vi "Tag Lookup_By Name.vi"(6 "Namespace":string, 8 "error in (no error)":errorcluster, 10 "Name":string) -> (0 "error out":errorcluster, 1 "found":bool, 2 "Tag Ref out":refnum<data-value>)   [LabVIEW 2020, in "Tag Engine Core.lvlib" / "Tag Core.lvclass"]
doc: "_SubVI_"
uses:
  Tag Core.lvclass
  Tag/Tag.lvclass
  Tag Core.lvclass/Tag Core.ctl
  <vilib>/Utility/error.llb/Error Cluster From Error Code.vi
  <vilib>/ErrorRing/Error Ring.xnode
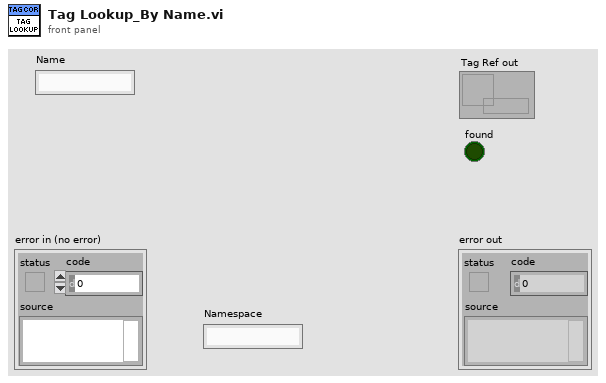
[diagram p1: front panel]
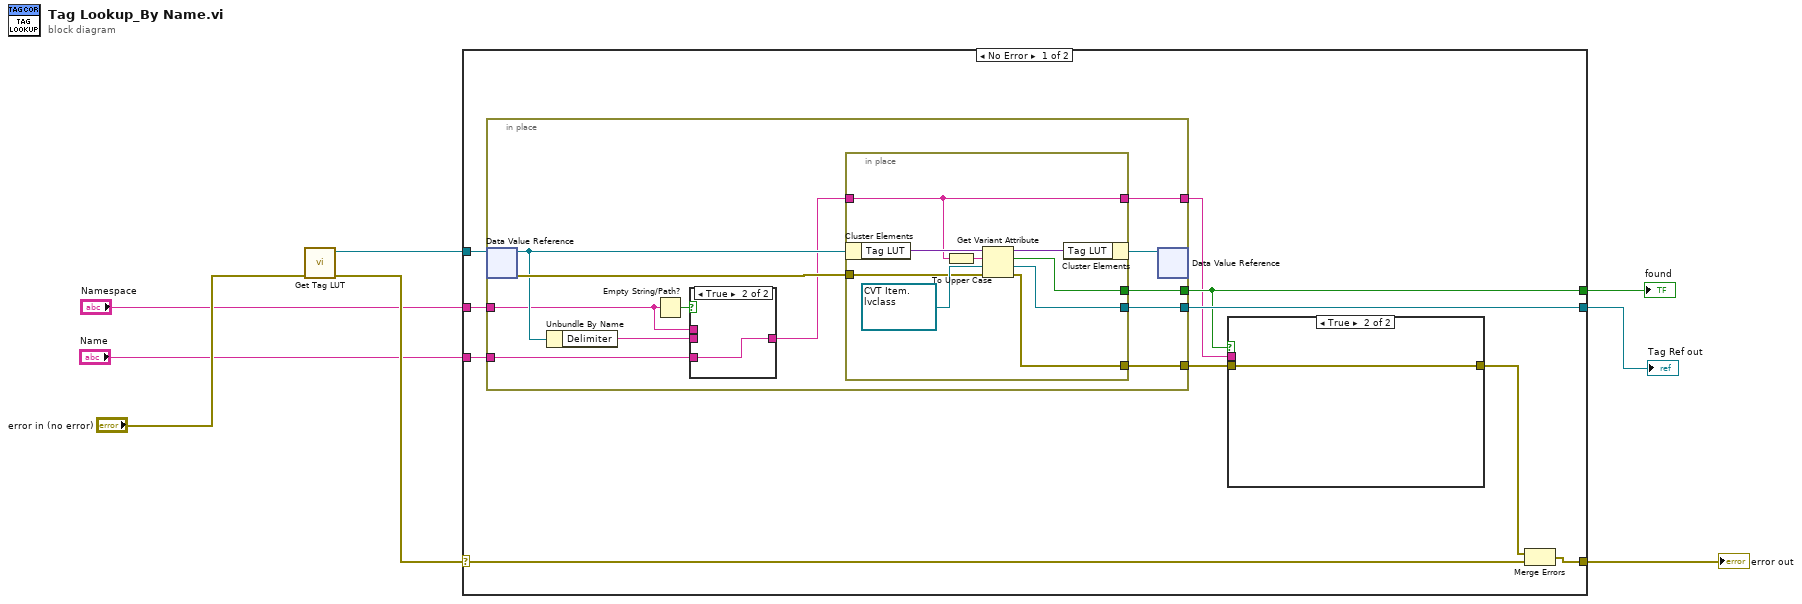
[diagram p0: block diagram]
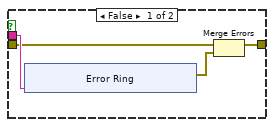
[diagram p2: hidden frame]
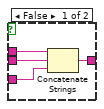
[diagram p3: hidden frame]
diagram:
  n1 = call "Get Tag LUT.vi"("error in (no error)"="error in (no error)") -> ("error out"=w4:errorcluster, "Tag LUT Out"=w3:refnum<data-value>)  [unwired: 9 in]
  n2 = case shown="No Error" w4 {
    selector: w4 -> [w13 w57]
    tunnel: [w14 w57] -> w8
    tunnel: w3 -> [w18 _]
    tunnel: [w17 _] -> w6
    tunnel: [w16 _] -> w7
    tunnel: "Name" -> [w10 _]
    tunnel: "Namespace" -> [w9 _]
    frame No Error {
      n3 = in-place {
        in-place-border: [w42] -> w17
        in-place-border: [w41] -> w16
        in-place-border: [w38] -> w15
        in-place-border: [w37] -> w11
        in-place-border: w10 -> [w33]
        in-place-border: w9 -> [w32]
        n4 = in-place-dvr #1(w18) -> (w36:refnum<class "Tag Core.lvclass">, w39:errorcluster)
        n5 = Unbundle By Name(w36) -> ("Delimiter"=w34:string)
        n6 = Empty String/Path?(string/path=w32) -> (empty?=w35:bool)
        n7 = case shown="False" w35 {
          tunnel: w32 -> [w46 _]
          tunnel: w33 -> [w45 w47]
          tunnel: [w44 w47] -> w31
          tunnel: w34 -> [w43 _]
          frame False {
            n8 = Concatenate Strings(w46, w43, w45) -> (w44:string)
          }
          frame True {
          }
        }
        n9 = in-place {
          in-place-border: w31 -> [w49]
          in-place-border: [w55] -> w42
          in-place-border: [w53] -> w41
          in-place-border: w39 -> [w51]
          in-place-border: [w50] -> w38
          in-place-border: [w49] -> w37
          n10 = in-place-cluster #2(w36) -> ("Tag LUT"=w56:variant)
          n11 = To Upper Case(1:w49) -> (0:w48:string)
          n12 = Get Variant Attribute(Variant=w56, name=w48, default value (empty Variant)=refnum<data-value> refnum ("CVT Item in"), error in=w51) -> (duplicate Variant=w54:variant, found=w53:bool, value=w55:refnum<data-value>, error out=w50:errorcluster)
          n13 = in-place-cluster #2("Tag LUT"=w54) -> (w40:refnum<class "Tag Core.lvclass">)
        }
        n14 = in-place-dvr #1(w40) -> ()  [unwired: 2 out]
      }
      n15 = case shown="False" w16 {
        tunnel: w15 -> [w21 w30]
        tunnel: [w19 w30] -> w12
        tunnel: w11 -> [w22 _]
        frame False {
          n16 = xnode "Error Ring"("parameter 0"=w22) -> ("error out"=w20:errorcluster)
          n17 = Merge Errors(w21, w20) -> (w19:errorcluster)
        }
        frame True {
        }
      }
      n18 = Merge Errors(w12, w13) -> (w14:errorcluster)
    }
    frame Error {
    }
  }
  "error out" <- w8
  "found" <- w7
  "Tag Ref out" <- w6
